vi "MySin.vi"(4 "x*y":dbl=5.0 format="%#_13g", 6 "AMP":dbl, 10 "Freq":dbl, 11 "Numeric 3":i32) -> (2 "Numeric":dbl, 3 "Numeric 2":dbl)   [LabVIEW 2025]
uses:
  <vilib>/ptbypt/NI_PtbyPt.lvlib
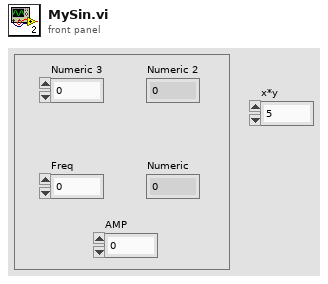
[diagram p1: front panel]
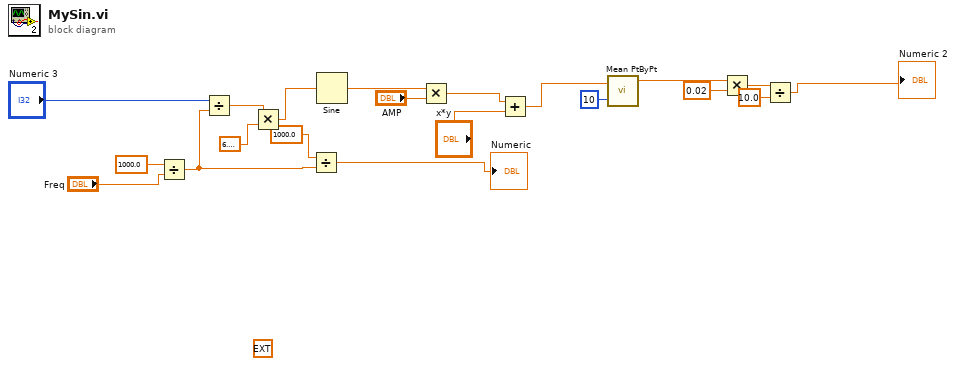
[diagram p0: block diagram]
diagram:
  (unwired) ext 0.0
  n1 = Divide(x=1000.0, y="Freq") -> (x/y=w15:dbl)
  n2 = Divide(x="Numeric 3", y=w15) -> (x/y=w11:dbl)
  n3 = Multiply(x=w11, y=6.283185307179586) -> (x*y=w17:dbl)
  n4 = Divide(x=1000.0, y=w15) -> (x/y=→"Numeric":dbl)
  n5 = Sine(x=w17) -> (sin(x)=w19:dbl)
  n6 = Multiply(x=w19, y="AMP") -> (x*y=w3:dbl)
  n7 = Add(x=w3, y="x*y") -> (x+y=w2:dbl)
  n8 = call <vilib>:"Mean PtByPt.vi"("x"=w2, "sample length"=10) -> ("mean"=w8:dbl)  [unwired: 2 in, 1 out]
  n9 = Multiply(x=w8, y=0.02) -> (x*y=w6:dbl)
  n10 = Divide(x=w6, y=10.0) -> (x/y=→"Numeric 2":dbl)
